vi "Get Status.vi"(8 "error in (no error)":errorcluster, 11 "FW Arduino Control in":refnum<class "FW Arduino Control.lvclass">) -> (0 "error out":errorcluster, 2 "FW Status":T1={"State"=enum."Move Complete", "Positions"=[], "Names"=[], "Notch"=[], "Moving"=[FALSE, FALSE]}, 3 "FW Arduino Control out":refnum<class "FW Arduino Control.lvclass">)   [LabVIEW 2024, in "FW Arduino Control.lvclass"]
uses:
  FW Arduino Control.lvclass
  FW cluster Status.ctl
  FW enum status.ctl
  Filter Wheel Object/Filter Wheel.lvclass
panel:
  out "Moving":bool[](array[boolean])
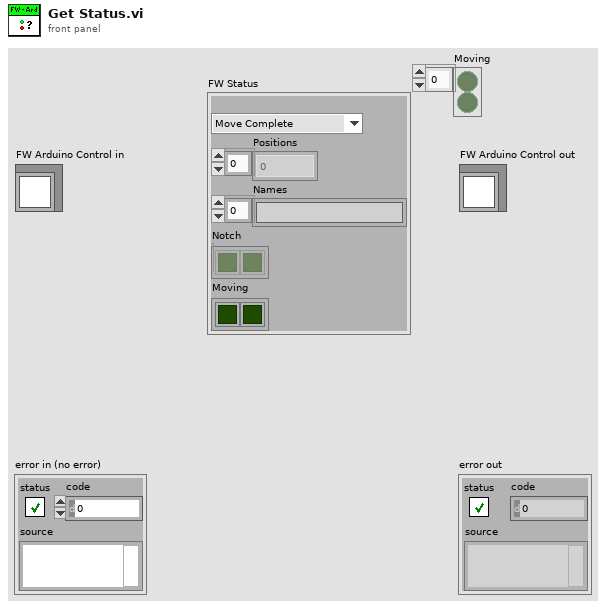
[diagram p1: front panel]
types:
  T1 = typedef "FW cluster Status.ctl" = cluster{"State":T2, "Positions":i32[], "Names":string[], "Notch":bool[], "Moving":bool[]}
  T2 = typedef "FW enum status.ctl" = enum16{"Initializing", "Moving", "Move Complete", "Error"}
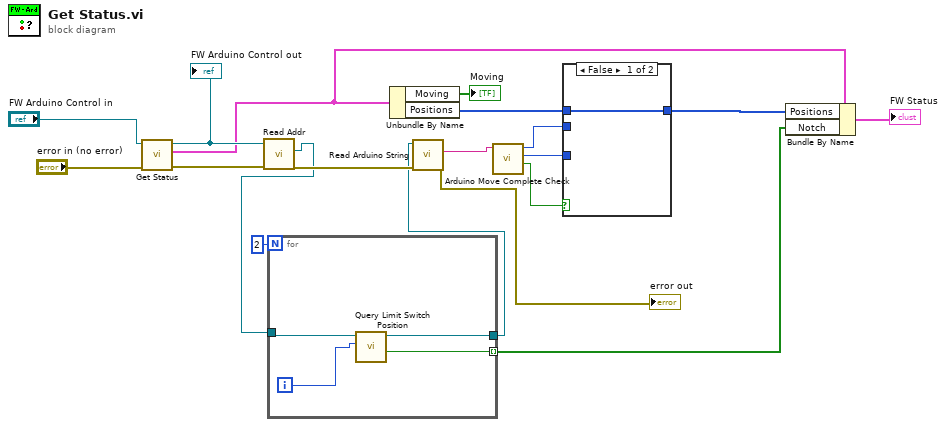
[diagram p0: block diagram]
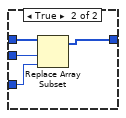
[diagram p2: hidden frame]
diagram:
  n1 = call-parent "Get Status.vi"("error in (no error)"="error in (no error)", "Filter Wheel in"="FW Arduino Control in") -> ("error out"=w13:errorcluster, "FW Status"=w1:T1, "Filter Wheel out"=w17:refnum<class "FW Arduino Control.lvclass">)  [unwired: 7 in]
  "FW Arduino Control out" <- w17
  n2 = call-dynamic "Read Addr.vi"("error in (no error)"=w13, "Filter Wheel in"=w17) -> ("error out"=w12:errorcluster, "Addr"=w6:refnum<visa-resource-name>)  [unwired: 7 in, 1 out]
  n3 = for {
    N: 2 -> [_]
    tunnel: w6 -> [w20]
    tunnel: [w23] -> w5
    tunnel: [w21] -> w4 mode=indexing
    i -> [w22]
    n4 = call "Query Limit Switch Position.vi"("motor (0:n-1)"=w22, "VISA resource name"=w20) -> ("At Switch?"=w21:bool, "reference out"=w23:refnum<visa-resource-name>)  [unwired: 5 in, 3 out]
  }
  n5 = Unbundle By Name(w1) -> ("Moving"=→"Moving":bool[], "Positions"=w16:i32[])
  n6 = call "Read Arduino String.vi"("error in (no error)"=w12, "reference"=w5) -> ("error out"=→"error out":errorcluster, "response"=w11:string)  [unwired: 7 in, 1 out]
  n7 = call "Arduino Move Complete Check.vi"("input string"=w11) -> ("Complete?"=w3:bool, "position"=w14:i32, "m"=w15:i32)  [unwired: 8 in]
  n8 = case shown="False" w3 {
    tunnel: w16 -> [w24 w28]
    tunnel: w15 -> [_ w27]
    tunnel: w14 -> [_ w26]
    tunnel: [w24 w25] -> w9
    frame False {
    }
    frame True {
      n9 = Replace Array Subset(array=w28, new element=w26, index=w27) -> (w25:i32[])
    }
  }
  n10 = Bundle By Name(cluster=w1, "Positions"=w9, "Notch"=w4) -> (→"FW Status":T1)
